vi "Obtain System Ref.vi"(8 "error in (no error)":errorcluster) -> (0 "error out":errorcluster, 3 "JKI SMO System":refnum<data-value>)   [LabVIEW 2013, in "Registry-SMO.lvclass"]
uses:
  Registry-SMO.lvclass
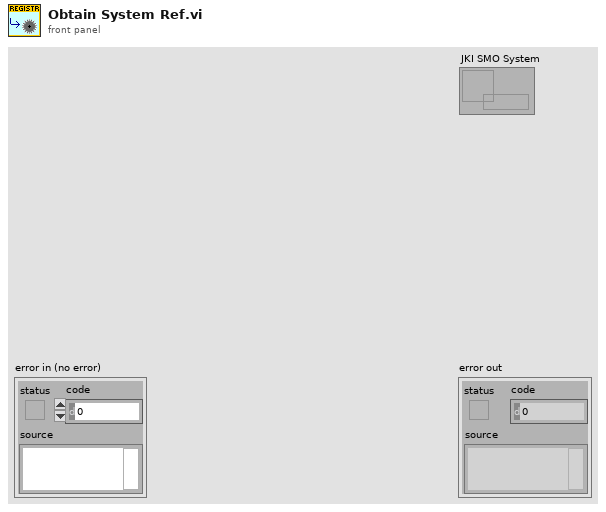
[diagram p1: front panel]
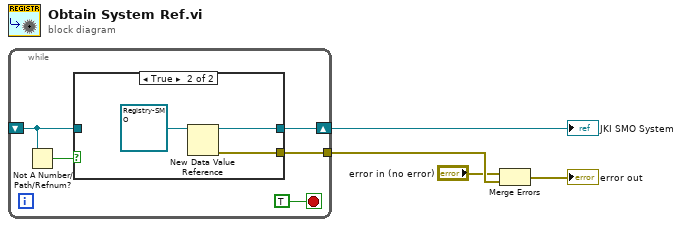
[diagram p0: block diagram]
diagram:
  n1 = while {
    shift-right: [w9] -> w4
    shift-left: _ -> [w6]
    tunnel: [w5] -> w3
    stop <- TRUE stop-if-true
    n2 = Not A Number/Path/Refnum?(number/path/refnum=w6) -> (NaN/Path/Refnum?=w7:bool)
    n3 = case shown="True" w7 {
      tunnel: [w10 w13] -> w9
      tunnel: w6 -> [w10 _]
      tunnel: [_ w11] -> w5
      frame False {
      }
      frame True {
        n4 = New Data Value Reference(data value=refnum<class "Registry-SMO.lvclass"> refnum ("JKI SMO System")) -> (data value reference=w13:refnum<data-value>, error out=w11:errorcluster)  [unwired: 1 in]
      }
    }
  }
  "JKI SMO System" <- w4
  n5 = Merge Errors("error in (no error)", w3) -> (→"error out":errorcluster)
